vi "PostMessage Master.vi"(0 "window refnum":T1, 2 "function":T2(ring)=enum."Start Screen Saver", 3 "error in (no error)":errorcluster) -> (5 "dup window refnum":T1, 7 "error out":errorcluster)   [LabVIEW 2023, in "WINUTIL.lvlib"]
doc: "This VI acts as a \"Master\" for various VIs that use the LVPostMessage function in the LVWUTIL.DLL library. This is basically just the PostMessage API function with a WM_SYSCOMMAND message, but also does some additional checking for the existance of the targeted window."
uses:
  WINUTIL.lvlib
  Window Refnum.ctl
  LVWUtil32.dll
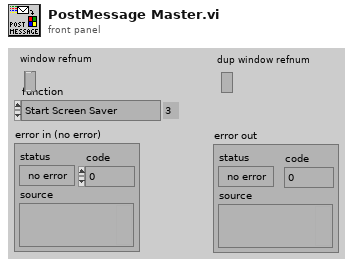
[diagram p1: front panel]
types:
  T1 = typedef "WINUTIL.lvlib/Window Refnum.ctl" = refnum<k1>
  T2 = enum8{"Maximize Window", "Minimize Window", "Show Task List", "Start Screen Saver", "Quit Application"}
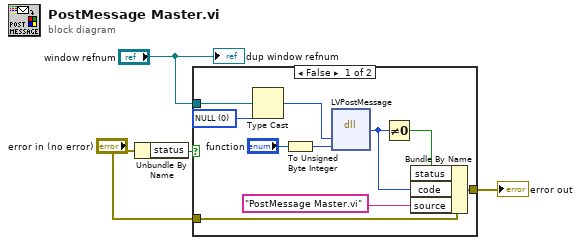
[diagram p0: block diagram]
diagram:
  n1 = Unbundle By Name("error in (no error)") -> ("status"=w4:bool)
  n2 = case shown="False" w4 {
    tunnel: "error in (no error)" -> [w13 w15]
    tunnel: [w10 w15] -> w2
    tunnel: "window refnum" -> [w5 _]
    frame False {
      w6 = u32 0 items=["NULL"]
      n3 = Type Cast(type=w6, x=w5) -> (*(type *) &x=w7:u32)
      n4 = To Unsigned Byte Integer(number="function") -> (unsigned 8bit integer=w8:u8)
      n5 = dll-call lib="C:/Users/acasalen/Documents/LabVIEW Data/Projects/Reds-Auto-Clicker/Red's Auto Clicker/SubVIs/labview_win_util32_8.6/LVWUtil32.DLL" fn="LVPostMessage"("hWnd"=w7, "function"=w8) -> ("error code"=w11:i32)  [unwired: 5 in, 2 out]
      n6 = Not Equal To 0?(x=w11) -> (x != 0?=w12:bool)
      n7 = Bundle By Name(cluster=w13, "status"=w12, "code"=w11, "source"="PostMessage Master.vi") -> (w10:errorcluster)
    }
    frame True {
    }
  }
  "error out" <- w2
  "dup window refnum" <- "window refnum"
